vi "Get Config File Path.vi"(8 "error in (no error)":T1 caption="entrée d'erreur (pas d'erreur)") -> (0 "error out":T1 caption="sortie d'erreur", 3 "Chemin du fichier XML":path)   [LabVIEW 2020, in "Settings.lvlib"]
doc: "Obtient le chemin du fichier XML de paramètres. La fonction Répertoire de l'application est utilisée à cette fin. Pour en savoir plus sur comment Répertoire de l'application calcule son chemin, cliquez avec le bouton droit sur la fonction et sélectionnez Aide."
uses:
  Settings.lvlib
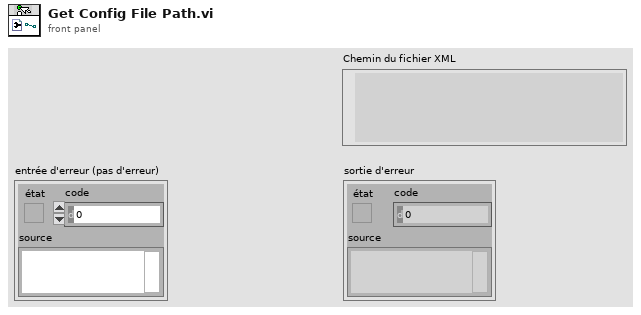
[diagram p1: front panel]
types:
  T1 = cluster{"état":bool, "code":i32, "source":string}
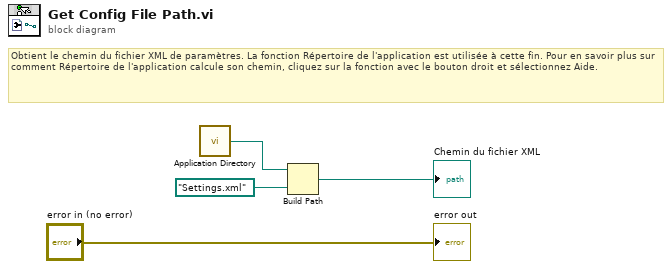
[diagram p0: block diagram]
diagram:
  # "Obtient le chemin du fichier XML de paramètres. La fonction Répertoire de l'application est utilisée à cette fin. Pour en savoir plus sur comment Répertoire de l'application calcule son chemin, cliquez sur la fonction avec le bouton droit et sélectionnez Aide."
  n1 = call <vilib>:"Application Directory.vi"() -> ("Application Directory"=w1:path)
  n2 = Build Path(base path=w1, name or relative path=path "Settings.xml" ("string")) -> (appended path=→"Chemin du fichier XML":path)
  "error out" <- "error in (no error)"
